vi "Initialize (Alternative).vi"(7 "Serial Configuration":T1={"Baud Rate"=9600, "Parity"=0, "Data Bits"=8, "Stop Bits"=10, "Flow Control"=0} {"Flow Control" items=["None", "XON/XOFF", "RTS/CTS", "XON/XOFF & RTS/CTS", "DTR/DSR", "XON/XOFF & DTR/DSR"]; "Stop Bits" items=["1.0"=10, "1.5"=15, "2.0"=20]; "Data Bits" items=["7"=7, "8"=8]; "Parity" items=["None", "Odd", "Even", "Mark", "Space"]; "Baud Rate" items=["300"=300, "600"=600, "1200"=1200, "2400"=2400, "4800"=4800, "9600"=9600, "19200"=19200]}, 8 "error in":errorcluster, 9 "Reset":bool=TRUE, 10 "ID Query":bool=TRUE, 11 "VISA resource name":refnum<visa-resource-name>) -> (0 "error out":errorcluster, 3 "VISA resource name out":refnum<visa-resource-name>)   [LabVIEW 2025]
doc: "Establishes communication with the instrument and optionally performs an instrument identification query and/or an instrument reset. It also places the instrument in a default state needed for other instrument driver operations. Therefore, call this VI before calling other instrument driver VIs for this instrument. Generally, you need to call the <b>Initialize</b> VI only once at the beginning of an application."
uses:
  <vilib>/Instr/_visa.llb/VISA Flush IO Buffer Mask.ctl
  <instrlib>/IT7800/IT7800.lvlib
panel:
  # "note: Alternative version with input buffer flush and synhronous R/W"
  # "EDIT: Change control description to remove example text for buses not supported."
  # "EDIT: Serial settings must match those on the physical instrument.  Review user's manual to determine the correct Flow Control protocol for the instrument.  \"None\" is the least robust option for this setting, and could lead to unreliable data transmission."
  # "EDIT: If your instrument does not support ID query or Reset, remove the ID Query or Reset control from the front panel and delete the case structure with the ID Query or Reset code from the block diagram."
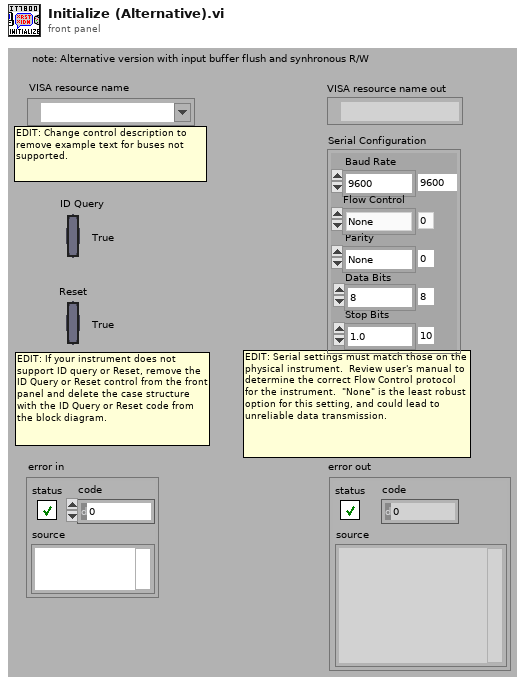
[diagram p1: front panel]
types:
  T1 = cluster{"Baud Rate":u32, "Parity":u16, "Data Bits":u16, "Stop Bits":u16, "Flow Control":u16}
  T2 = typedef "VISA Flush IO Buffer Mask.ctl" = u16
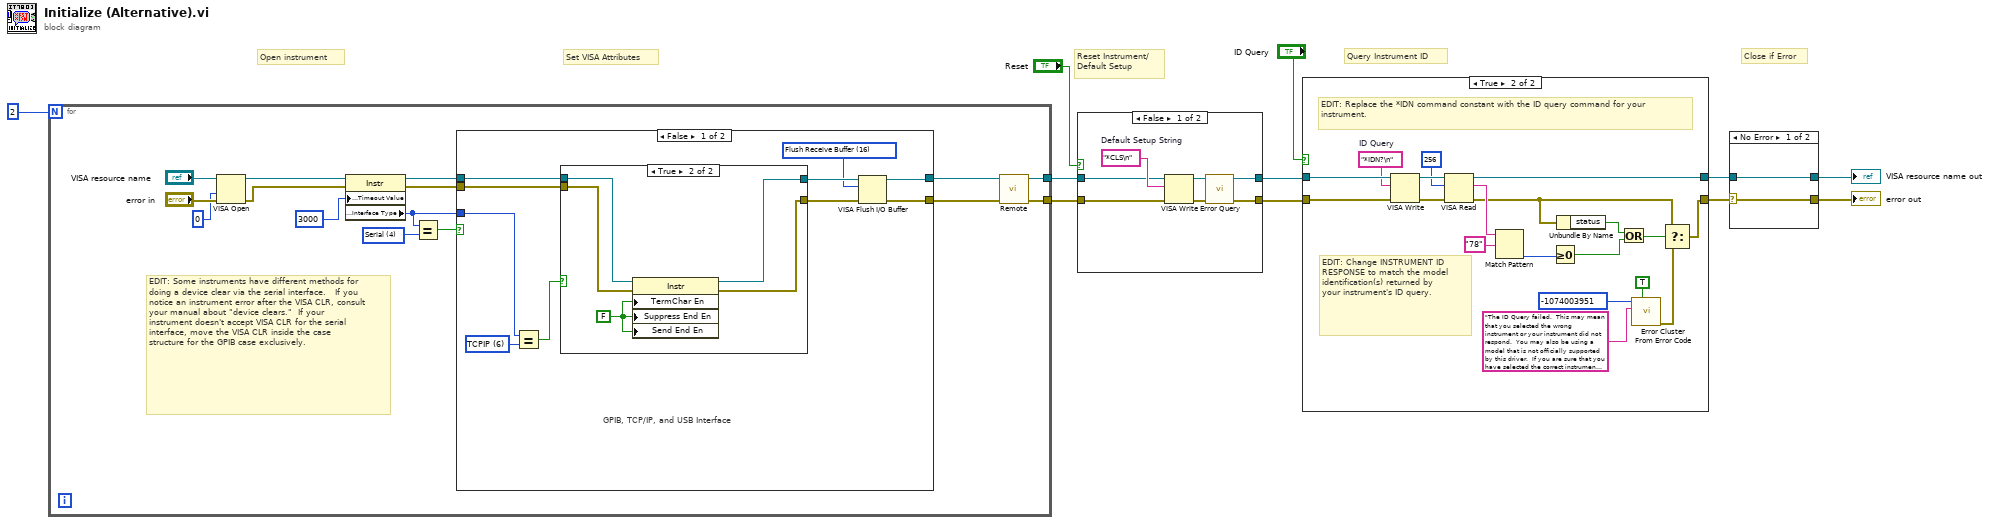
[diagram p0: block diagram]
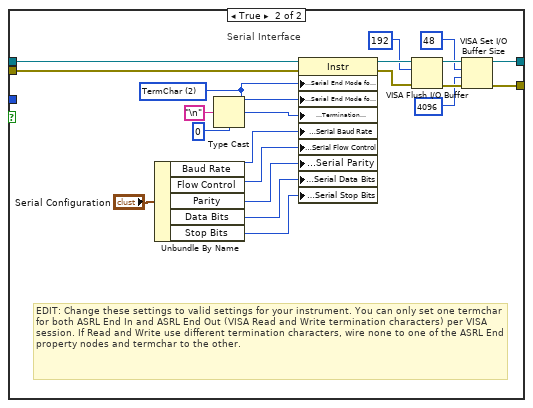
[diagram p3: hidden frame]
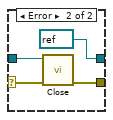
[diagram p4: hidden frame]
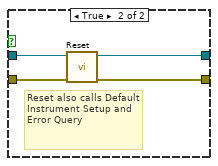
[diagram p5: hidden frame]
diagram:
  # "Set VISA Attributes"
  # "Close if Error"
  # "Query Instrument ID"
  # "Reset Instrument/\nDefault Setup"
  # "Open instrument"
  n1 = for {
    N: 2 -> [_]
    tunnel: [w24] -> w6
    tunnel: [w23] -> w5
    w17 = u16 4 items=["GPIB"=1, "VXI"=2, "GPIB-VXI"=3, "Serial"=4, "PXI"=5, "TCPIP"=6, "USB"=7] ("Interface Information:Interface Type")
    # "EDIT: Some instruments have different methods for doing a device clear via the serial interface.   If you notice an instrument error after the VISA CLR, consult your manual about \"device clears.\"  If your instrument doesn't accept VISA CLR for the serial interface, move the VISA CLR inside the case  structure for the GPIB case exclusively."
    n2 = VISA Open(access mode=u32 0, error in (no error)="error in", VISA resource name="VISA resource name") -> (VISA resource name=w13:refnum<visa-resource-name>, error out=w12:errorcluster)  [unwired: 2 in]
    n3 = property class="Instr"(reference=w13, error in=w12, "General Settings:Timeout Value"=u32 3000) -> (reference out=w19:refnum<visa-resource-name>, error out=w18:errorcluster, "Interface Information:Interface Type"=w15:u16)
    n4 = Equal?(x=w15, y=w17) -> (x = y?=w14:bool)
    n5 = case shown="False" w14 {
      tunnel: [w29 w61] -> w26
      tunnel: [w28 w58] -> w25
      tunnel: w19 -> [w33 w63]
      tunnel: w18 -> [w32 w64]
      tunnel: w15 -> [w34 _]
      frame False {
        w27 = T2 16 items=["Flush Receive Buffer"=16, "Write Transmit Buffer to Device"=32, "Flush Receive Buffer (No I/O)"=64, "Flush Transmit Buffer"=128] ("Mask")
        w35 = u16 6 items=["GPIB"=1, "VXI"=2, "GPIB-VXI"=3, "Serial"=4, "PXI"=5, "TCPIP"=6, "USB"=7] ("Interface Information:Interface Type")
        # "GPIB, TCP/IP, and USB Interface"
        n6 = Equal?(x=w34, y=w35) -> (x = y?=w36:bool)
        n7 = case shown="True" w36 {
          tunnel: [w38 w43] -> w31
          tunnel: [w37 w42] -> w30
          tunnel: w33 -> [w38 w41]
          tunnel: w32 -> [w37 w40]
          frame False {
          }
          frame True {
            w39 = FALSE
            n8 = property class="Instr"(reference=w41, error in=w40, "TermChar En"=w39, "Suppress End En"=w39, "Send End En"=w39) -> (reference out=w43:refnum<visa-resource-name>, error out=w42:errorcluster)
          }
        }
        n9 = VISA Flush I/O Buffer(VISA resource name=w31, mask (16)=w27, error in (no error)=w30) -> (VISA resource name out=w29:refnum<visa-resource-name>, error out=w28:errorcluster)
      }
      frame True {
        w51 = u16 2 items=["None", "LastBit", "TermChar"] ("Serial Settings:Serial End Mode for Reads")
        # "EDIT: Change these settings to valid settings for your instrument. You can only set one termchar for both ASRL End In and ASRL End Out (VISA Read and Write termination characters) per VISA session. If Read and Write use different termination characters, wire none to one of the ASRL End property nodes and termchar to the other."
        # "Serial Interface"
        n10 = Unbundle By Name("Serial Configuration") -> ("Baud Rate"=w49:u32, "Flow Control"=w45:u16, "Parity"=w47:u16, "Data Bits"=w48:u16, "Stop Bits"=w44:u16)
        n11 = Type Cast(type=u8 0, x="\n" ("Line Feed Constant")) -> (*(type *) &x=w50:u8)
        n12 = property class="Instr"(reference=w63, error in=w64, "Serial Settings:Serial End Mode for Reads"=w51, "Serial Settings:Serial End Mode for Writes"=w51, "Message Based Settings:Termination Character"=w50, "Serial Settings:Serial Baud Rate"=w49, "Serial Settings:Serial Flow Control"=w45, "Serial Settings:Serial Parity"=w47, "Serial Settings:Serial Data Bits"=w48, "Serial Settings:Serial Stop Bits"=w44) -> (reference out=w57:refnum<visa-resource-name>, error out=w60:errorcluster)
        n13 = VISA Flush I/O Buffer(VISA resource name=w57, mask (16)=u16 192, error in (no error)=w60) -> (VISA resource name out=w62:refnum<visa-resource-name>, error out=w59:errorcluster)
        n14 = VISA Set I/O Buffer Size(VISA resource name=w62, mask (16)=u16 48, size (4096)=u32 4096 ("size (0)"), error in (no error)=w59) -> (VISA resource name out=w61:refnum<visa-resource-name>, error out=w58:errorcluster)
      }
    }
    n15 = call <instrlib>:"Remote.vi"("error in"=w25, "VISA resource name"=w26) -> ("error out"=w23:errorcluster, "VISA resource name out"=w24:refnum<visa-resource-name>)  [unwired: 8 in]
  }
  n16 = case shown="False" "Reset" {
    tunnel: w5 -> [w67 w72]
    tunnel: [w70 w75] -> w3
    tunnel: w6 -> [w68 w73]
    tunnel: [w71 w74] -> w4
    frame False {
      w69 = "*CLS\n"  # Default Setup String
      n17 = VISA Write(VISA resource name=w68, write buffer=w69, error in (no error)=w67) -> (VISA resource name out=w65:refnum<visa-resource-name>, error out=w66:errorcluster)  [unwired: 1 out]
      n18 = call <instrlib>:"Error Query.vi"("error in"=w66, "VISA resource name"=w65) -> ("error out"=w70:errorcluster, "VISA resource name out"=w71:refnum<visa-resource-name>)  [unwired: 6 in, 2 out]
    }
    frame True {
      # "Reset also calls Default Instrument Setup and Error Query"
      n19 = call <instrlib>:"Reset.vi"("error in"=w72, "VISA resource name"=w73) -> ("error out"=w75:errorcluster, "VISA resource name out"=w74:refnum<visa-resource-name>)  [unwired: 8 in]
    }
  }
  n20 = case shown="True" "ID Query" {
    tunnel: [w76 w96] -> w1
    tunnel: [w77 w93] -> w2
    tunnel: w4 -> [w77 w94]
    tunnel: w3 -> [w76 w95]
    frame False {
    }
    frame True {
      w87 = "*IDN?\n"  # ID Query
      # "EDIT: Replace the *IDN command constant with the ID query command for your instrument."
      # "EDIT: Change INSTRUMENT ID RESPONSE to match the model identification(s) returned by your instrument's ID query."
      n21 = VISA Write(VISA resource name=w94, write buffer=w87, error in (no error)=w95) -> (VISA resource name out=w91:refnum<visa-resource-name>, error out=w90:errorcluster)  [unwired: 1 out]
      n22 = VISA Read(VISA resource name=w91, byte count=u32 256, error in (no error)=w90) -> (VISA resource name out=w93:refnum<visa-resource-name>, read buffer=w92:string, error out=w81:errorcluster)  [unwired: 1 out]
      n23 = Match Pattern(string=w92, regular expression="78") -> (offset past match=w82:i32)  [unwired: 1 in, 3 out]
      n24 = Greater Or Equal To 0?(x=w82) -> (x >= 0?=w79:bool)
      n25 = Unbundle By Name(w81) -> ("status"=w80:bool)
      n26 = Or(x=w80, y=w79) -> (x .or. y?=w78:bool)
      n27 = call <vilib>:"Error Cluster From Error Code.vi"("show call chain? (False)"=TRUE, "error message (\"\")"="The ID Query failed.  This may mean that you selected the wrong instrument or your instrument did not respond.  You may also be using a model that is not officially supported by this driver.  If you are sure that you have selected the correct instrument and it is responding, try disabling the ID Query." ("Source (VI Name)"), "error code (0)"=-1074003951 ("Code")) -> ("error out"=w86:errorcluster)  [unwired: 6 in]
      n28 = Select(t=w81, s=w78, f=w86) -> (s? t:f=w96:errorcluster)
    }
  }
  n29 = case shown="No Error" w1 {
    selector: w1 -> [w97 w100]
    tunnel: w2 -> [w98 w101]
    tunnel: [w98 refnum<visa-resource-name> refnum ("VISA resource name out")] -> w9
    tunnel: [w97 w102] -> w8
    frame No Error {
    }
    frame Error {
      n30 = call <instrlib>:"Close.vi"("error in"=w100, "VISA resource name"=w101) -> ("error out"=w102:errorcluster)  [unwired: 9 in]
    }
  }
  "VISA resource name out" <- w9
  "error out" <- w8
